vi "_number_of_devices.vi"(8 "error in (no error)":errorcluster, 11 "UV-VIS_AVANTES in":refnum<class "UV-VIS_AVANTES.lvclass">) -> (0 "error out":errorcluster, 2 "# spectrometers":i32, 3 "UV-VIS_AVANTES out":refnum<class "UV-VIS_AVANTES.lvclass">)   [LabVIEW 2020, in "UV-VIS_AVANTES.lvclass"]
uses:
  UV-VIS_AVANTES.lvclass
  C:/dev/TRANCON/Classes/Detector/Detector.lvclass
  Detector.lvclass/Detector.ctl
  Detector.lvclass
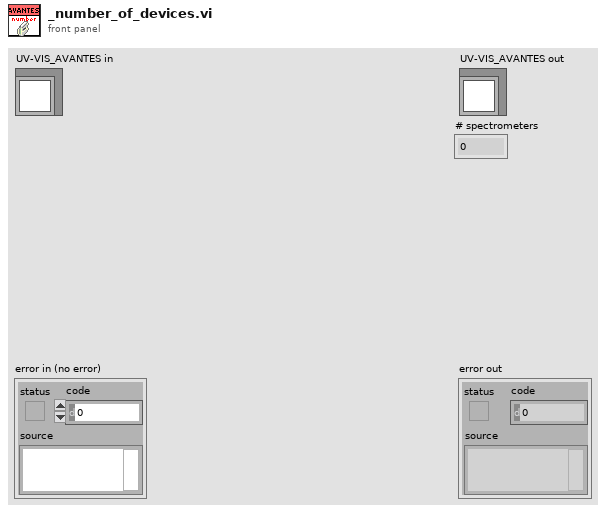
[diagram p1: front panel]
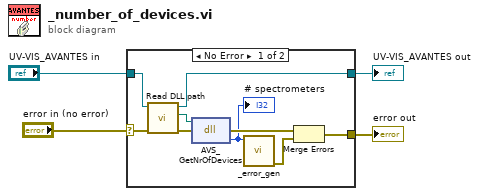
[diagram p0: block diagram]
diagram:
  n1 = case shown="No Error" "error in (no error)" {
    selector: "error in (no error)" -> [w12 w15]
    tunnel: [w5 w15] -> w3
    tunnel: [w11 w14] -> w1
    tunnel: "UV-VIS_AVANTES in" -> [w13 w14]
    frame No Error {
      n2 = call "Read DLL path.vi"("error in (no error)"=w12, "Detector in"=w13) -> ("error out"=w9:errorcluster, "DLL path"=w10:path, "Detector out"=w11:refnum<class "UV-VIS_AVANTES.lvclass">)  [unwired: 7 in]
      n3 = dll-call lib="C:/AvaSpecX64-DLL_9.4/examples/LabView/LabViewSingleChan/avaspec.dll" fn="AVS_GetNrOfDevices"(path in=w10, error in=w9) -> (error out=w7:errorcluster, "return type"=w6:i32)  [unwired: 1 in, 1 out]
      "# spectrometers" <- w6
      n4 = call "_error_gen.vi"("return type"=w6) -> ("error out"=w8:errorcluster)  [unwired: 10 in]
      n5 = Merge Errors(w7, w8) -> (w5:errorcluster)
    }
    frame Error {
    }
  }
  "error out" <- w3
  "UV-VIS_AVANTES out" <- w1
